vi "name.vi"(8 "error in (no error)":errorcluster, 11 "ChickenBurger in":refnum<class "ChickenBurger.lvclass">) -> (0 "error out":errorcluster, 2 "name":string, 3 "ChickenBurger out":refnum<class "ChickenBurger.lvclass">)   [LabVIEW 2016, in "ChickenBurger.lvclass"]
uses:
  ChickenBurger.lvclass
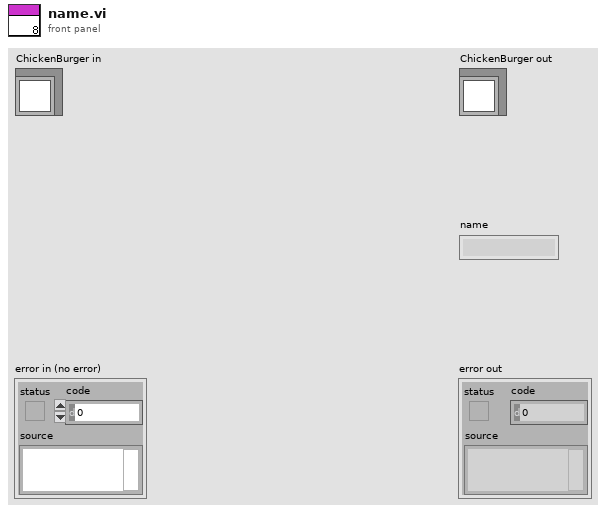
[diagram p1: front panel]
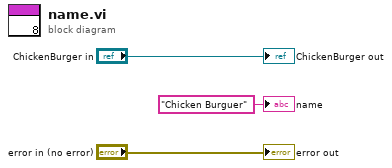
[diagram p0: block diagram]
diagram:
  "error out" <- "error in (no error)"
  "ChickenBurger out" <- "ChickenBurger in"
  "name" <- "Chicken Burguer" ("name")
